vi "higher caller.vi"() -> (3 "LabVIEW Text":string)   [LabVIEW 2013]
panel:
  in  "hb":bool=TRUE
  in  "h ts":timestamp=timestamp(3523589884.3778296 s since 1904-01-01)
  in  "h num":dbl=34.0
  in  "h str":string="asdassasd"
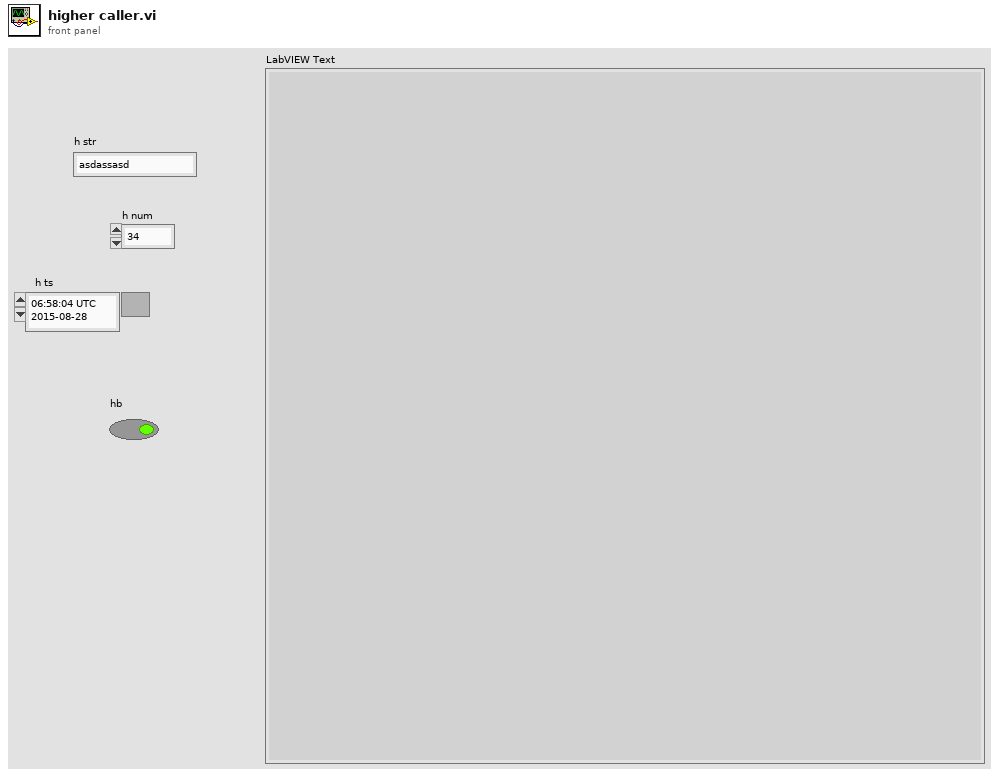
[diagram p1: front panel]
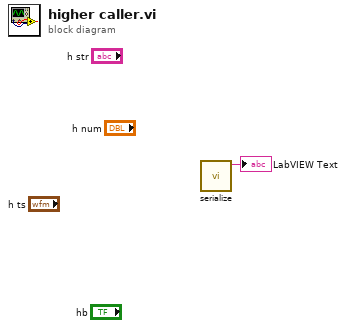
[diagram p0: block diagram]
diagram:
  n1 = call "serialize.vi"() -> ("LabVIEW Text"=→"LabVIEW Text":string)  [unwired: 10 in, 1 out]
